vi "Configure.vi"(8 "error in (no error)":errorcluster, 11 "Galvo in":refnum<class "ImagingModeSPIM.lvclass">) -> (0 "error out":errorcluster, 2 "cancelled?":bool=TRUE, 3 "Galvo out":refnum<class "ImagingModeSPIM.lvclass">)   [LabVIEW 2012, in "ImagingModeSPIM.lvclass"]
doc: "The configure method configures the details for the RabbitMQ connection. \n\nIn the derived class, make a call to the parent for setting these parameters."
uses:
  ImagingModeSPIM.lvclass
  Controls/number of channels.ctl
  <vilib>/Utility/miscctls.llb/LVPointTypeDef.ctl
  ImagingModeSPIM.lvclass/ImagingModeSPIM.ctl
  <vilib>/Distrio/Murmex/Murmex/Murmex.lvclass
panel:
  in  "Tab Control":enum32{"Waveform", "Task"}(tab)
  in  "Number of channels":T1
  in  "Samples/channel":i32=1000
  in  "Sampling rate":dbl=10000.0 format="%#_6e"
  in  "physical channels":tag
  in  "minimum value":dbl[unit]=-10.0 format="%0.2f"
  in  "maximum value":dbl[unit]=10.0 format="%0.2f"
  in  "button::cancel":bool
  in  "button::ok":bool
  in  "button::configure murmex":bool
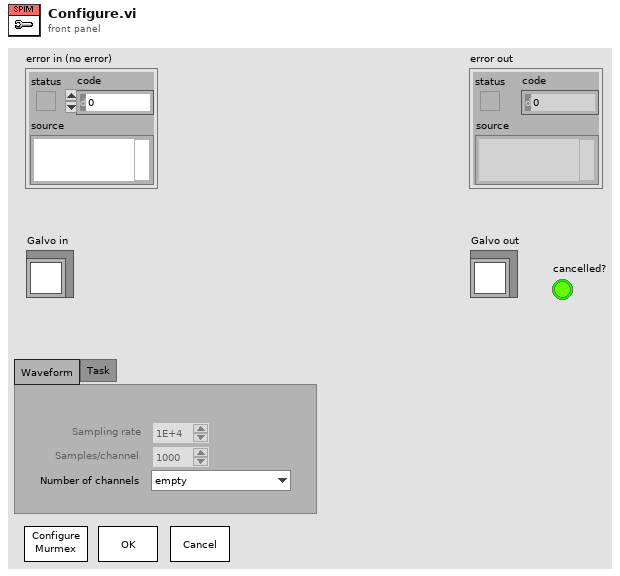
[diagram p1: front panel]
types:
  T1 = typedef "ImagingModeSPIM.lvclass/number of channels.ctl" = enum16{"empty", "double sided + PC", "double sided + WFS"}
  T2 = typedef "LVPointTypeDef.ctl" = cluster{"Horizontal":i16, "Vertical":i16}
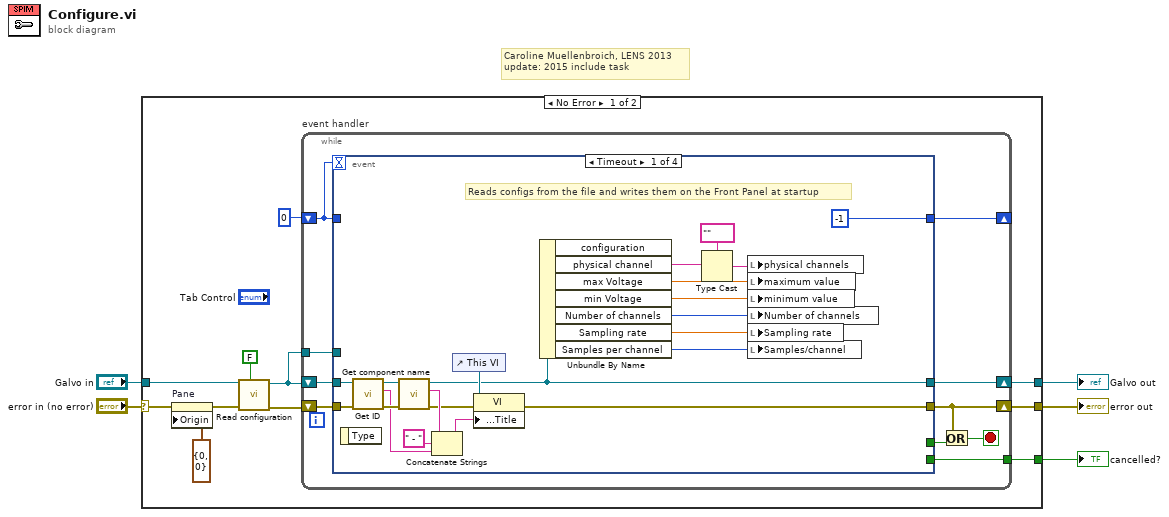
[diagram p0: block diagram]
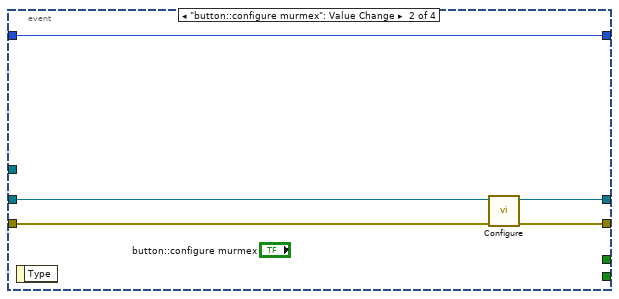
[diagram p2: hidden frame]
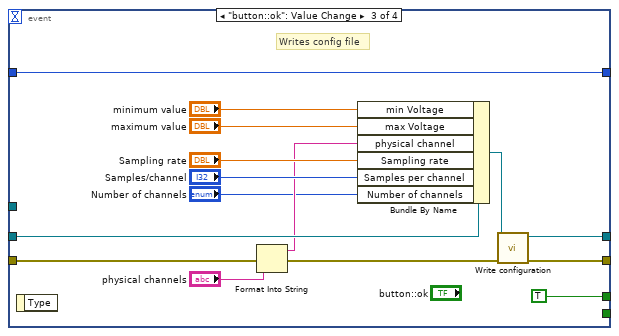
[diagram p3: hidden frame]
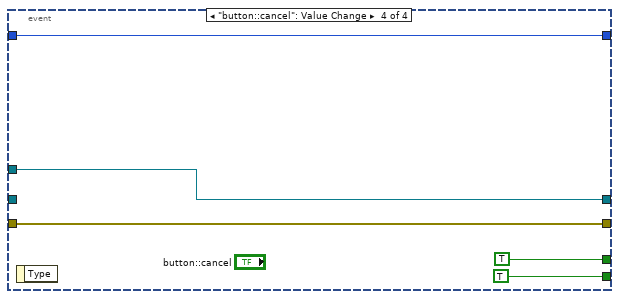
[diagram p4: hidden frame]
diagram:
  # "Caroline Muellenbroich, LENS 2013\nupdate: 2015 include task"
  n1 = case shown="No Error" "error in (no error)" {
    selector: "error in (no error)" -> [w10 w74]
    tunnel: [w15 _] -> w5
    tunnel: [w14 w73] -> w4
    tunnel: [w13 w74] -> w3
    tunnel: "Galvo in" -> [w11 w73]
    frame No Error {
      n2 = property on="Pane" class="Pane"(error in=w10, "Origin"=T2 {"Horizontal"=0, "Vertical"=0}) -> (error out=w8:errorcluster)  [unwired: 1 in, 1 out]
      n3 = call-dynamic "Read configuration.vi"("force loading?"=FALSE, "error in (no error)"=w8, "Galvo in"=w11) -> ("error out"=w7:errorcluster, "Galvo out"=w6:refnum<class "ImagingModeSPIM.lvclass">)  [unwired: 7 in]
      n4 = while "event handler" {
        shift-right: [w26] -> _
        shift-left: 0 -> [w17]
        shift-right: [w23] -> w14
        shift-left: w6 -> [w24]
        shift-right: [w22] -> w13
        shift-left: w7 -> [w25]
        tunnel: [w19] -> w15
        tunnel: w6 -> [w18]
        stop <- w20 stop-if-true
        n5 = event shown="[0] Timeout" {
          selector: _ -> [_ _ _ _]
          dyn-events: _ -> [_ _ _ _]
          timeout: w17 -> [_ _ _ _]
          tunnel: w17 -> [_ w48 w62 w69]
          tunnel: [-1 w48 w62 w69] -> w26
          tunnel: w25 -> [w42 w51 w58 w72]
          tunnel: w24 -> [w46 w52 w65 _]
          tunnel: [w34 w50 w67 w68] -> w23
          tunnel: [w33 w49 w66 w72] -> w22
          tunnel: [_ _ TRUE ("force loading?") TRUE ("force loading?")] -> w21
          tunnel: [_ _ _ TRUE ("force loading?")] -> w19
          tunnel: w18 -> [_ _ _ w68]
          event Timeout {
            # "Reads configs from the file and writes them on the Front Panel at startup"
            n6 = event-data() -> ()  [unwired: 1 in, 1 out]
            n7 = call <vilib>:"Get ID.vi"("error in (no error)"=w42, "Murmex in"=w46) -> ("error out"=w41:errorcluster, "component id"=w37:string, "Murmex out"=w40:refnum<class "ImagingModeSPIM.lvclass">)  [unwired: 7 in]
            n8 = call <vilib>:"Get component name.vi"("error in (no error)"=w41, "Murmex in"=w40) -> ("error out"=w35:errorcluster, "component name"=w36:string, "Murmex out"=w34:refnum<class "ImagingModeSPIM.lvclass">)  [unwired: 7 in]
            n9 = Concatenate Strings(w36, " - " ("string"), w37) -> (w38:string)
            n10 = control-ref of="This VI"() -> (w43:refnum<vi>)
            n11 = property class="VI"(reference=w43, error in=w35, "Front Panel.Title"=w38) -> (error out=w33:errorcluster)  [unwired: 1 out]
            n12 = Unbundle By Name(w34) -> ("physical channel"=w29:string, "max Voltage"=w30:dbl[unit], "min Voltage"=w31:dbl[unit], "Number of channels"=w32:T1, "Sampling rate"=w45:dbl, "Samples per channel"=w44:i32)  [unwired: 1 out]
            n13 = Type Cast(type=tag "" ("physical channels"), x=w29) -> (*(type *) &x=w27:tag)
            n14 = local write "physical channels"(w27) -> ()
            n15 = local write "maximum value"(w30) -> ()
            n16 = local write "minimum value"(w31) -> ()
            n17 = local write "Number of channels"(w32) -> ()
            n18 = local write "Sampling rate"(w45) -> ()
            n19 = local write "Samples/channel"(w44) -> ()
          }
          event "button::configure murmex": Value Change {
            n20 = event-data() -> ()  [unwired: 1 in, 1 out]
            n21 = call-parent "Configure.vi"("error in (no error)"=w51, "Murmex in"=w52) -> ("error out"=w49:errorcluster, "Murmex out"=w50:refnum<class "ImagingModeSPIM.lvclass">)  [unwired: 7 in, 1 out]
          }
          event "button::ok": Value Change {
            # "Writes config file"
            n22 = event-data() -> ()  [unwired: 1 in, 1 out]
            n23 = Format Into String(error in=w58, "physical channels") -> (resulting string=w59:string, error out=w57:errorcluster)  [unwired: 2 in]
            n24 = Bundle By Name(cluster=w65, "min Voltage"="minimum value", "max Voltage"="maximum value", "physical channel"=w59, "Sampling rate"="Sampling rate", "Samples per channel"="Samples/channel", "Number of channels"="Number of channels") -> (w64:refnum<class "ImagingModeSPIM.lvclass">)
            n25 = call-dynamic "Write configuration.vi"("error in (no error)"=w57, "Galvo in"=w64) -> ("error out"=w66:errorcluster, "Galvo out"=w67:refnum<class "ImagingModeSPIM.lvclass">)  [unwired: 8 in]
          }
          event "button::cancel": Value Change {
            n26 = event-data() -> ()  [unwired: 1 in, 1 out]
          }
        }
        n27 = Or(x=w22, y=w21) -> (x .or. y?=w20:bool)
      }
    }
    frame Error {
    }
  }
  "error out" <- w3
  "Galvo out" <- w4
  "cancelled?" <- w5
